vi "JoystickDeadband.vi"(8 "Deadband %":dbl, 11 "Joystick Value":dbl) -> (3 "Joystick Value":dbl)   [LabVIEW 2018]
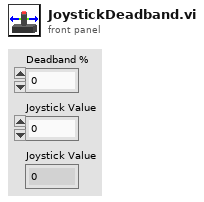
[diagram p1: front panel]
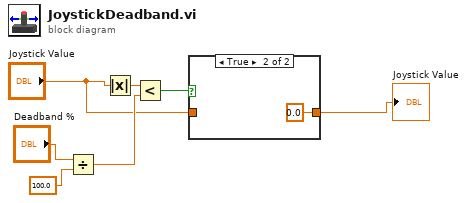
[diagram p0: block diagram]
diagram:
  n1 = Divide(x="Deadband %", y=100.0) -> (x/y=w5:dbl)
  n2 = Absolute Value(x="Joystick Value") -> (abs(x)=w4:dbl)
  n3 = Less?(x=w4, y=w5) -> (x < y?=w3:bool)
  n4 = case shown="True" w3 {
    tunnel: [w8 0.0 ("Joystick Value")] -> w2
    tunnel: "Joystick Value" -> [w8 _]
    frame False {
    }
    frame True {
    }
  }
  "Joystick Value" <- w2
